vi "Get Modal Sampling Frequency.vi"(1 "XY Data In":cluster{"Yo":dbl, "Xo":timestamp}[](array[cluster])) -> (0 "Measured Fs":dbl)   [LabVIEW 2014]
uses:
  <vilib>/Analysis/baseanly.llb/Unimode.vi
  <vilib>/Analysis/NI_AALBase.lvlib
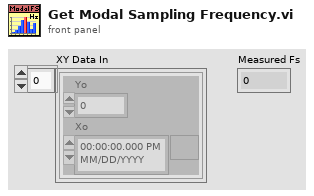
[diagram p1: front panel]
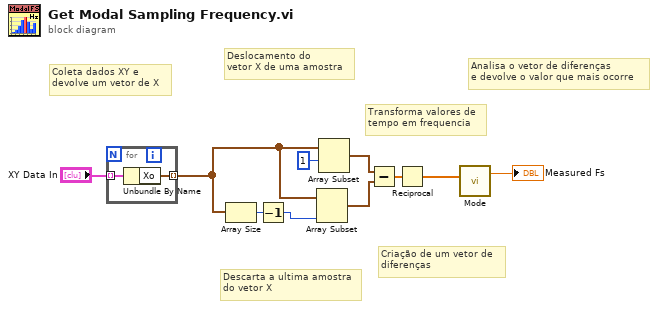
[diagram p0: block diagram]
diagram:
  # "Transforma valores de\ntempo em frequencia"
  # "Descarta a ultima amostra\ndo vetor X"
  # "Analisa o vetor de diferenças\ne devolve o valor que mais ocorre"
  # "Criação de um vetor de\ndiferenças"
  # "Deslocamento do \nvetor X de uma amostra"
  # "Coleta dados XY e \ndevolve um vetor de X"
  n1 = for {
    tunnel: [w12] -> w7 mode=indexing
    tunnel: "XY Data In" -> [w11] mode=indexing
    n2 = Unbundle By Name(w11) -> ("Xo"=w12:timestamp)
  }
  n3 = Array Size(array=w7) -> (size(s)=w1:i32)
  n4 = Decrement(x=w1) -> (x-1=w3:i32)
  n5 = Array Subset(array=w7, length=w3) -> (w4:timestamp[])  [unwired: 1 in]
  n6 = Array Subset(array=w7, index=1) -> (w5:timestamp[])  [unwired: 1 in]
  n7 = Subtract(x=w5, y=w4) -> (x-y=w6:dbl[])
  n8 = Reciprocal(x=w6) -> (1/x=w9:dbl[])
  n9 = call-poly <vilib>:"Mode.vi"("X"=w9) -> ("mode"=→"Measured Fs":dbl)  [unwired: 1 in, 1 out]
